vi "Handle Last Ack Core.vi"(4 "error in (no error)":errorcluster, 6 "Last Ack":refnum<class "Last Ack.lvclass">, 7 "Root Actor in":refnum<class "Root Actor.lvclass">) -> (0 "error out":errorcluster, 3 "Root Actor out":refnum<class "Root Actor.lvclass">)   [LabVIEW 2020, in "Nested Actor.lvlib" / "Root Actor.lvclass"]
doc: "(<B>Filename</B>: Actor Framework.lvlib:Actor.lvclass:Handle Last Ack Core.vi)\n\nDefines how the caller actor responds to the Last Ack message from a nested actor. The Last Ack message is the final message a nested actor sends to its caller before it shuts down. The message contains information about the final state of the nested actor.\n\nBy default, this method does nothing except return any error the nested actor sent. A descendant class may override this method to define behavior."
uses:
  Root Actor.lvclass
  <vilib>/ActorFramework/LastAck/Last Ack.lvclass
  Root Actor.lvclass/Root Actor.ctl
  <vilib>/ActorFramework/Actor/Actor.lvclass
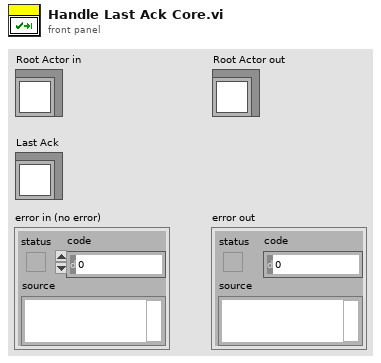
[diagram p1: front panel]
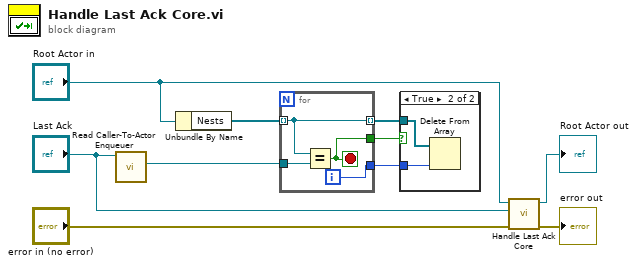
[diagram p0: block diagram]
diagram:
  n1 = call <vilib>:"Read Caller-To-Actor Enqueuer.vi"("Last Ack"="Last Ack") -> ("Caller-to-Actor Enqueuer"=w4:refnum<class "Message Enqueuer.lvclass">)  [unwired: 10 in]
  n2 = Unbundle By Name("Root Actor in") -> ("Nests"=w5:refnum<class "Message Enqueuer.lvclass">[])
  n3 = for {
    tunnel: w5 -> [w12] mode=indexing
    tunnel: w4 -> [w14]
    tunnel: [w13] -> w3
    tunnel: [w12] -> w2 mode=indexing
    tunnel: [w11] -> w1
    i -> [w11]
    stop <- w13 stop-if-true
    n4 = Equal?(x=w12, y=w14) -> (x = y?=w13:bool)
  }
  n5 = case shown="True" w3 {
    tunnel: w2 -> [_ w16]
    tunnel: w1 -> [_ w15]
    frame False {
    }
    frame True {
      n6 = Delete From Array(array=w16, index=w15) -> ()  [unwired: 1 in, 2 out]
    }
  }
  n7 = call-parent "Handle Last Ack Core.vi"("error in (no error)"="error in (no error)", "Last Ack"="Last Ack", "Actor in"="Root Actor in") -> ("error out"=→"error out":errorcluster, "Actor out"=→"Root Actor out":refnum<class "Root Actor.lvclass">)  [unwired: 3 in]
